vi "ValidateError.vi"(8 "error in (no error)":errorcluster) -> (0 "error out":errorcluster, 3 "NoError?":bool)   [LabVIEW 2017]
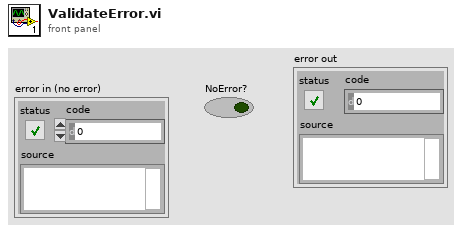
[diagram p1: front panel]
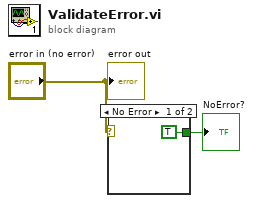
[diagram p0: block diagram]
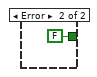
[diagram p2: hidden frame]
diagram:
  n1 = case shown="No Error" "error in (no error)" {
    tunnel: [TRUE FALSE] -> w2
    frame No Error {
    }
    frame Error {
    }
  }
  "NoError?" <- w2
  "error out" <- "error in (no error)"
